vi "main_qsm.vi"() -> ()   [LabVIEW 2015]
uses:
  queue_state_&_argument (Array).vi
  <vilib>/Utility/error.llb/Error Cluster From Error Code.vi
  queue_state_&_argument (Single).vi
  <vilib>/ErrorRing/Error Ring.xnode
panel:
  in  "Run Test 2":bool
  in  "Run Test 1":bool
  in  "Stop Button":bool
  # "State Machine with Arguments"
  # "Improving string-based_State_Machine"
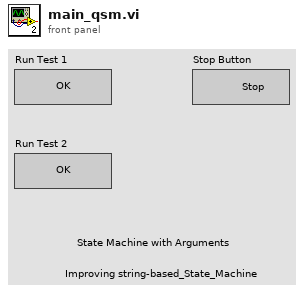
[diagram p1: front panel]
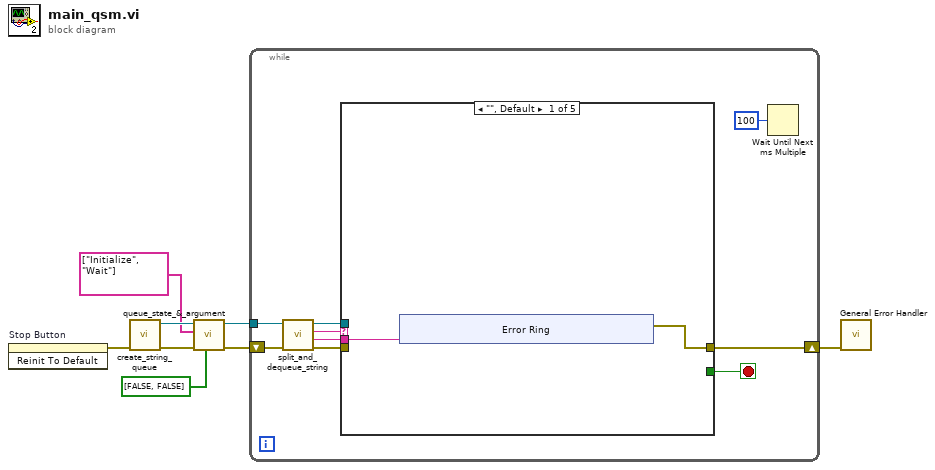
[diagram p0: block diagram]
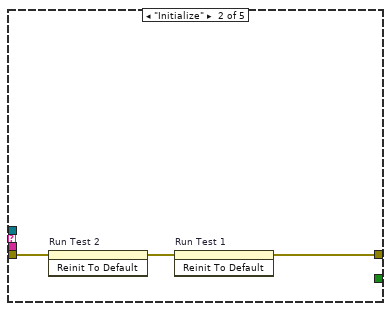
[diagram p2: hidden frame]
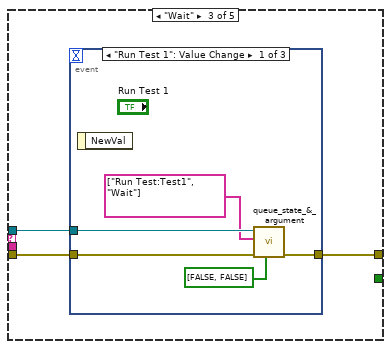
[diagram p3: hidden frame]
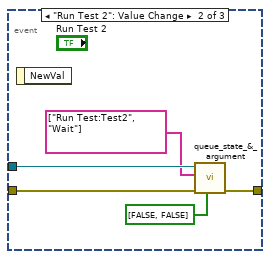
[diagram p4: hidden frame]
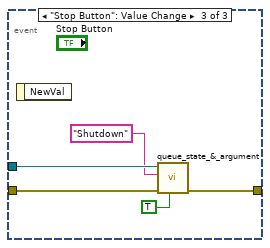
[diagram p5: hidden frame]
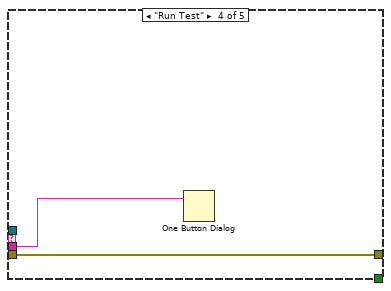
[diagram p6: hidden frame]
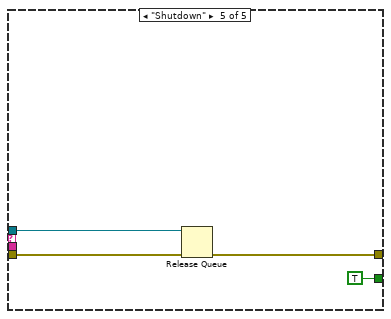
[diagram p7: hidden frame]
diagram:
  n1 = invoke on="Stop Button" class="Bool" method="Reinit To Default"() -> (error out=w7:errorcluster)  [unwired: 3 in, 2 out]
  n2 = call "create_string_queue.vi"("error in (no error)"=w7) -> ("error out"=w5:errorcluster, "Queue out"=w4:refnum<queue>)  [unwired: 9 in]
  n3 = call-poly "queue_state_&_argument.vi"("Priority? Array"=bool[] [FALSE, FALSE], "error in (no error)"=w5, "state:argument array"=string[] ["Initialize", "Wait"], "Queue in"=w4) -> ("error out"=w6:errorcluster, "Queue out"=w3:refnum<queue>)  [unwired: 6 in]
  n4 = while {
    shift-right: [w16] -> w8
    shift-left: w6 -> [w10]
    tunnel: w3 -> [w9]
    stop <- w15 stop-if-true
    n5 = call "split_and_dequeue_string.vi"("error in (no error)"=w10, "Queue in"=w9) -> ("error out"=w13:errorcluster, "argument"=w11:string, "state"=w12:string, "Queue out"=w14:refnum<queue>)  [unwired: 6 in]
    n6 = case shown="\"\", Default" w12 {
      tunnel: w13 -> [_ w29 w32 w49 w52]
      tunnel: [w18 w27 w31 w49 w50] -> w16
      tunnel: [_ _ _ _ TRUE] -> w15
      tunnel: w14 -> [_ _ w30 _ w51]
      tunnel: w11 -> [w19 _ _ w48 _]
      frame "", Default {
        n7 = xnode "Error Ring"("parameter 0"=w19) -> ("error out"=w18:errorcluster)
      }
      frame "Initialize" {
        n8 = invoke on="Run Test 2" class="Bool" method="Reinit To Default"(error in=w29) -> (error out=w28:errorcluster)  [unwired: 2 in, 2 out]
        n9 = invoke on="Run Test 1" class="Bool" method="Reinit To Default"(error in=w28) -> (error out=w27:errorcluster)  [unwired: 2 in, 2 out]
      }
      frame "Wait" {
        n10 = event shown="[0] \"Run Test 1\": Value Change" {
          selector: _ -> [_ _ _]
          dyn-events: _ -> [_ _ _]
          timeout: _ -> [_ _ _]
          tunnel: w32 -> [w36 w42 w46]
          tunnel: [w35 w41 w47] -> w31
          tunnel: w30 -> [w34 w40 w45]
          event "Run Test 1": Value Change {
            n11 = event-data() -> ()  [unwired: 1 in, 1 out]
            n12 = call-poly "queue_state_&_argument.vi"("Priority? Array"=bool[] [FALSE, FALSE], "error in (no error)"=w36, "state:argument array"=string[] ["Run Test:Test1", "Wait"], "Queue in"=w34) -> ("error out"=w35:errorcluster)  [unwired: 6 in, 1 out]
          }
          event "Run Test 2": Value Change {
            n13 = event-data() -> ()  [unwired: 1 in, 1 out]
            n14 = call-poly "queue_state_&_argument.vi"("Priority? Array"=bool[] [FALSE, FALSE], "error in (no error)"=w42, "state:argument array"=string[] ["Run Test:Test2", "Wait"], "Queue in"=w40) -> ("error out"=w41:errorcluster)  [unwired: 6 in, 1 out]
          }
          event "Stop Button": Value Change {
            n15 = event-data() -> ()  [unwired: 1 in, 1 out]
            n16 = call-poly "queue_state_&_argument.vi"("Priority? (F)"=TRUE, "error in (no error)"=w46, "state:argument"="Shutdown", "Queue in"=w45) -> ("error out"=w47:errorcluster)  [unwired: 6 in, 1 out]
          }
        }
      }
      frame "Run Test" {
        n17 = One Button Dialog(message=w48) -> ()  [unwired: 1 in, 1 out]
      }
      frame "Shutdown" {
        n18 = Release Queue(queue=w51, error in (no error)=w52) -> (error out=w50:errorcluster)  [unwired: 1 in, 2 out]
      }
    }
    n19 = Wait Until Next ms Multiple(millisecond multiple=u32 100) -> ()  [unwired: 1 out]
  }
  n20 = call <vilib>:"General Error Handler.vi"("error in (no error)"=w8) -> ()  [unwired: 10 in, 5 out]
